vi "Initialize.vi"(8 "error in (no error)":errorcluster, 11 "State in":T1={"State"=enum."Idle", "Start Time"=timestamp(0 s since 1904-01-01), "Configuration"={"Cycle Period"=0.0, "PID 2 Parameters"={"Input Device"=enum."4-20mA", "Output Device"=enum."Default", "Setpoint"=0.0, "PID gains"={"proportional gain (Kc)"=0.0, "integral time (Ti, min)"=0.0, "derivative time (Td, min)"=100.0}, "output range"={"output low"=0.0, "output high"=1.0}}, "Manual Entry"=0.0, "Auto?"=TRUE, "4-20mA Input Settings"={"Input Channel "=0}, "4-20mA Out Settings"={"Output DAQ Task"=""}, "Input Channel Tag Name "=""}, "Current Time"=timestamp(0 s since 1904-01-01), "PID 1 Parameters"={"Setpoint"=0.0, "PID gains"={"proportional gain (Kc)"=1.0, "integral time (Ti, min)"=0.01, "derivative time (Td, min)"=0.0}}, "First Iteration"=FALSE, "Data"={"4-20mA Input"=0.0, "PID 2 Process Variable"=0.0, "PID 2 Output"=0.0, "4-20mA Output"=0.0}, "Process Name"="", "Pump On?"=enum."Off", "Input Error"=FALSE, "Output Error"=FALSE, "Log Started"=FALSE, "Current Setpoint"=0.0} {"Configuration"."PID 2 Parameters"."output range"."output low" format="%.2f"; "Configuration"."PID 2 Parameters"."output range"."output high" min=0.0 max=100.0 format="%.2f"; "Configuration"."PID 2 Parameters"."PID gains"."derivative time (Td, min)" format="%.3f"; "Configuration"."PID 2 Parameters"."PID gains"."integral time (Ti, min)" format="%.3f"; "Configuration"."PID 2 Parameters"."PID gains"."proportional gain (Kc)" format="%.3f"; "PID 1 Parameters"."PID gains"."derivative time (Td, min)" format="%.3f"; "PID 1 Parameters"."PID gains"."integral time (Ti, min)" format="%.3f"; "PID 1 Parameters"."PID gains"."proportional gain (Kc)" format="%.3f"}) -> (0 "error out":errorcluster, 1 "Pump Initialized":bool, 3 "State out":T1={"State"=enum."Idle", "Start Time"=timestamp(0 s since 1904-01-01), "Configuration"={"Cycle Period"=0.0, "PID 2 Parameters"={"Input Device"=enum."4-20mA", "Output Device"=enum."Default", "Setpoint"=0.0, "PID gains"={"proportional gain (Kc)"=0.0, "integral time (Ti, min)"=0.0, "derivative time (Td, min)"=100.0}, "output range"={"output low"=0.0, "output high"=1.0}}, "Manual Entry"=0.0, "Auto?"=TRUE, "4-20mA Input Settings"={"Input Channel "=0}, "4-20mA Out Settings"={"Output DAQ Task"=""}, "Input Channel Tag Name "=""}, "Current Time"=timestamp(0 s since 1904-01-01), "PID 1 Parameters"={"Setpoint"=0.0, "PID gains"={"proportional gain (Kc)"=1.0, "integral time (Ti, min)"=0.01, "derivative time (Td, min)"=0.0}}, "First Iteration"=FALSE, "Data"={"4-20mA Input"=0.0, "PID 2 Process Variable"=0.0, "PID 2 Output"=0.0, "4-20mA Output"=0.0}, "Process Name"="", "Pump On?"=enum."Off", "Input Error"=FALSE, "Output Error"=FALSE, "Log Started"=FALSE, "Current Setpoint"=0.0} {"Configuration"."PID 2 Parameters"."output range"."output low" format="%.2f"; "Configuration"."PID 2 Parameters"."output range"."output high" min=0.0 max=100.0 format="%.2f"; "Configuration"."PID 2 Parameters"."PID gains"."derivative time (Td, min)" format="%.3f"; "Configuration"."PID 2 Parameters"."PID gains"."integral time (Ti, min)" format="%.3f"; "Configuration"."PID 2 Parameters"."PID gains"."proportional gain (Kc)" format="%.3f"; "PID 1 Parameters"."PID gains"."derivative time (Td, min)" format="%.3f"; "PID 1 Parameters"."PID gains"."integral time (Ti, min)" format="%.3f"; "PID 1 Parameters"."PID gains"."proportional gain (Kc)" format="%.3f"})   [LabVIEW 2018, in "4-20mA Module.lvlib" / "4-20mA Module Engine.lvlib"]
uses:
  4-20mA Module Engine.lvlib
  State Cluster.ctl
  State Enum.ctl
  Pressure Transmitter/Pressure Transmitter Device Settings.ctl
  Pressure Reg Module/Pressure Regulator Device Settings.ctl
  Measure Instrument/PID 1 Parameters Cluster.ctl
  Tag VIs/Tag FGV Operation Enum.ctl
  Shared Variables/Dynamic Shared Variables.lvlib
  Pressure Transmitter/Pressure Transmitter Library.lvlib
  Pressure Reg Module/Pressure Regulator Library.lvlib
panel:
  # "Instrument Settings"
  # "Instrument Settings"
  # "Instrument Settings"
  # "Instrument Settings"
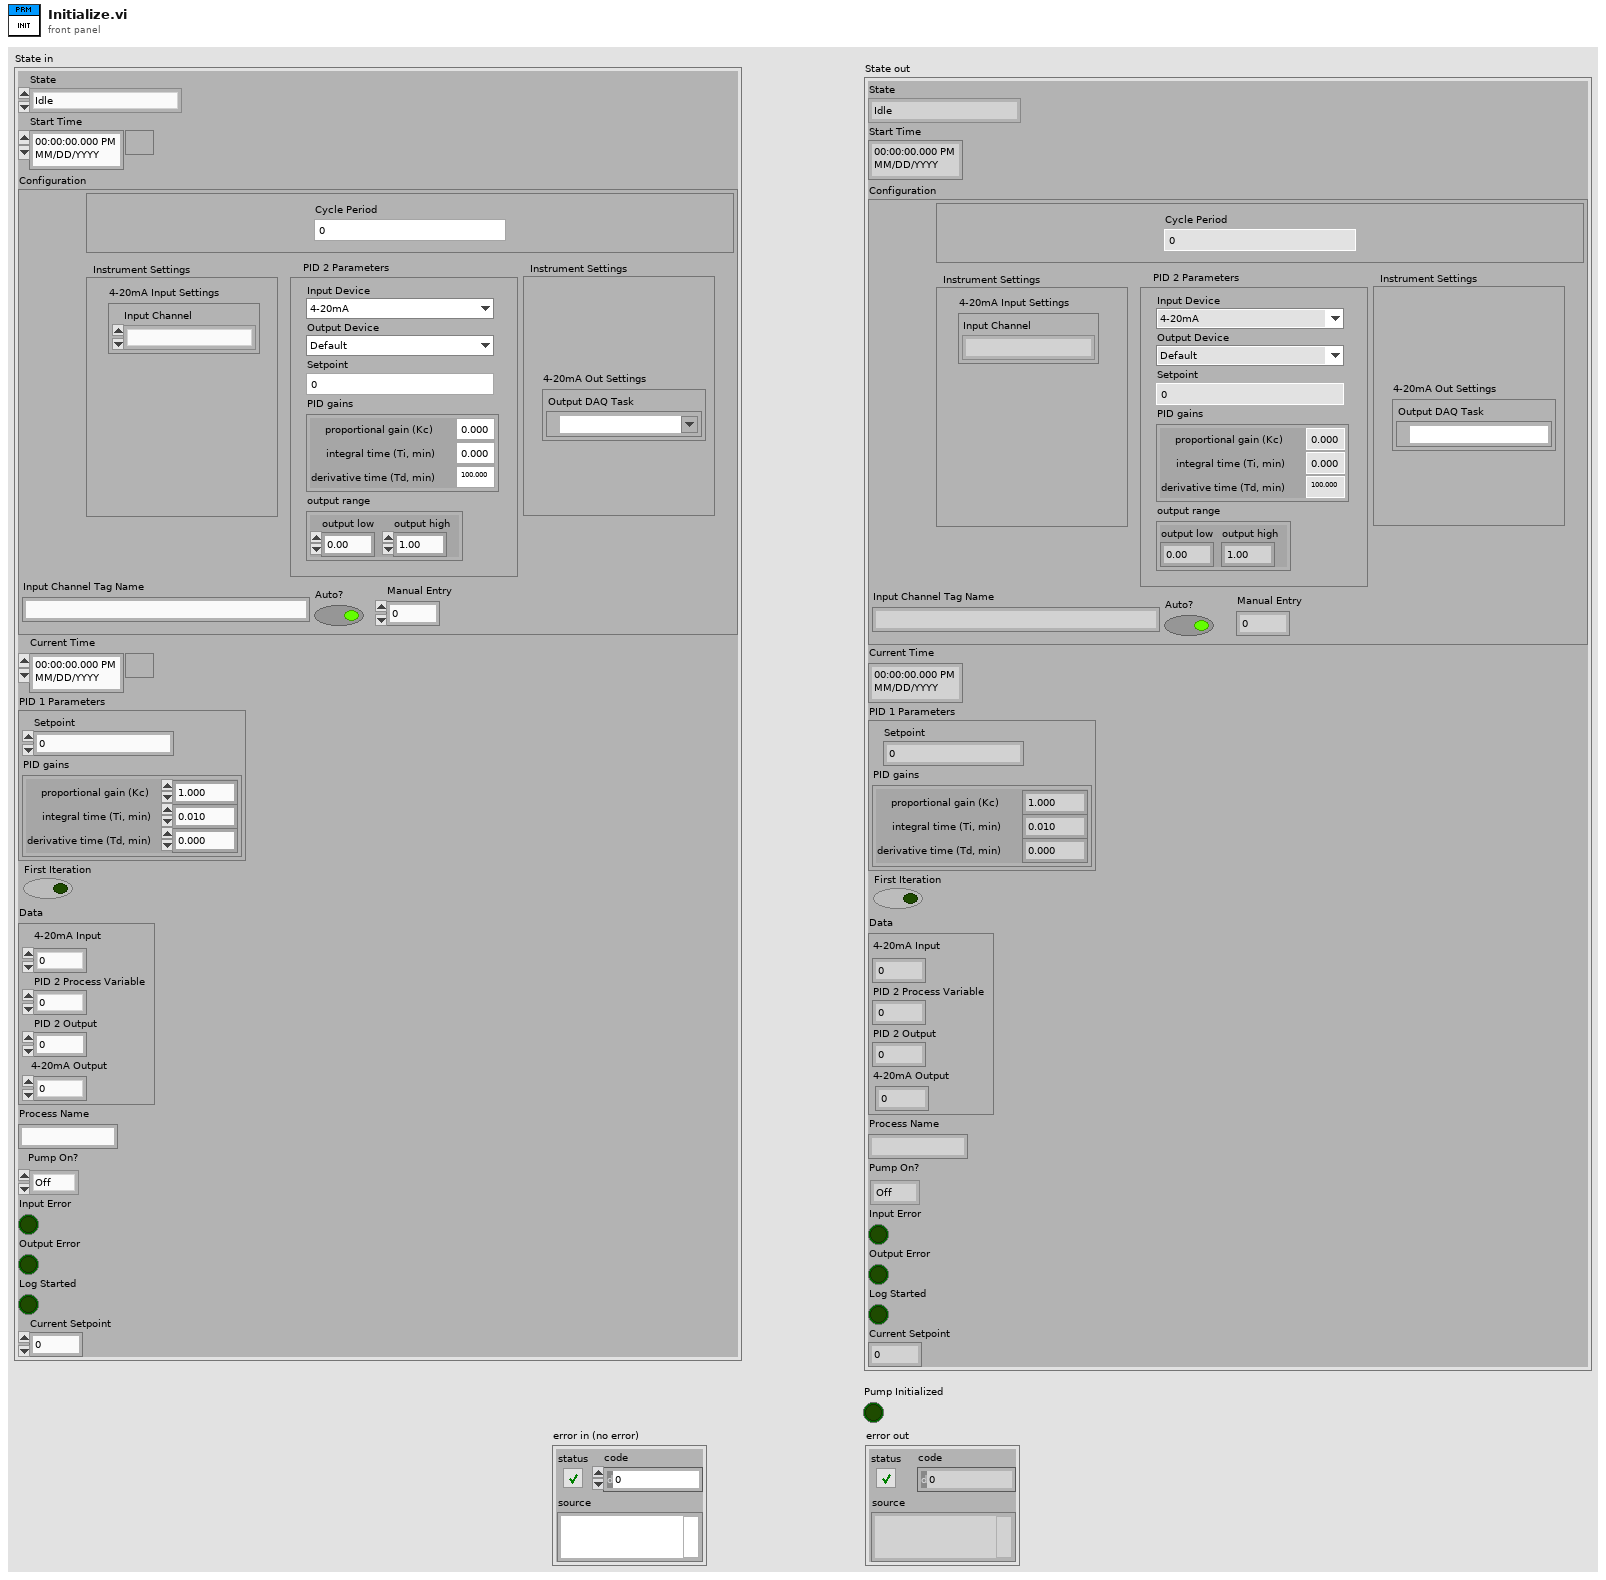
[diagram p1: front panel]
types:
  T1 = typedef "4-20mA Module.lvlib/4-20mA Module Engine.lvlib/State Cluster.ctl" = cluster{"State":T2, "Start Time":timestamp, "Configuration":cluster{"Cycle Period":dbl, "PID 2 Parameters":cluster{"Input Device":enum16{"Default", "4-20mA"}, "Output Device":enum16{"Default", "Equilibar Pressure Reg", "Flow Regulator"}, "Setpoint":dbl, "PID gains":cluster{"proportional gain (Kc)":dbl, "integral time (Ti, min)":dbl, "derivative time (Td, min)":dbl}, "output range":cluster{"output low":dbl, "output high":dbl}}, "Manual Entry":dbl, "Auto?":bool, "4-20mA Input Settings":T3, "4-20mA Out Settings":T4, "Input Channel Tag Name ":string}, "Current Time":timestamp, "PID 1 Parameters":T5, "First Iteration":bool, "Data":cluster{"4-20mA Input":dbl, "PID 2 Process Variable":dbl, "PID 2 Output":dbl, "4-20mA Output":dbl}, "Process Name":string, "Pump On?":enum16{"Off", "On", "Not Initialized"}, "Input Error":bool, "Output Error":bool, "Log Started":bool, "Current Setpoint":dbl}
  T2 = typedef "4-20mA Module.lvlib/4-20mA Module Engine.lvlib/State Enum.ctl" = enum16{"Measuring", "Idle", "Paused"}
  T3 = typedef "Pressure Transmitter Library.lvlib/Pressure Transmitter Device Settings.ctl" = cluster{"Input Channel ":u16}
  T4 = typedef "Pressure Regulator Library.lvlib/Pressure Regulator Device Settings.ctl" = cluster{"Output DAQ Task":refnum<k21>}
  T5 = typedef "PID 1 Parameters Cluster.ctl" = cluster{"Setpoint":dbl, "PID gains":cluster{"proportional gain (Kc)":dbl, "integral time (Ti, min)":dbl, "derivative time (Td, min)":dbl}}
  T6 = typedef "Tag FGV Operation Enum.ctl" = enum16{"Init", "Set Notification Queue", "Create Tag", "Commit", "Write Tag (Numeric)", "Write Tag (Boolean)", "Read All Tags", "Read One Tag", "Delete Tag Category", "Set Alarm Parameters (Numeric)", "Set Alarm Parameters (Boolean)", "Enable All Alarms", "Disable All Alarms", "Delete All Tags", "Read Alarms", "Ack Alarm", "Read Alarm Parameters (Numeric)", "Read Alarm Parameters (Boolean)"}
  T7 = typedef "4-20mA Module.lvlib/4-20mA Module Tag Names Cluster.ctl" = cluster{"4-20mA Input":string, "PID 2 Out Tag":string, "4-20mA Output":string, "Input Device Tag":string, "Output Device Tag":string}
  T8 = enum16{"Default", "Equilibar Pressure Reg", "Flow Regulator"}
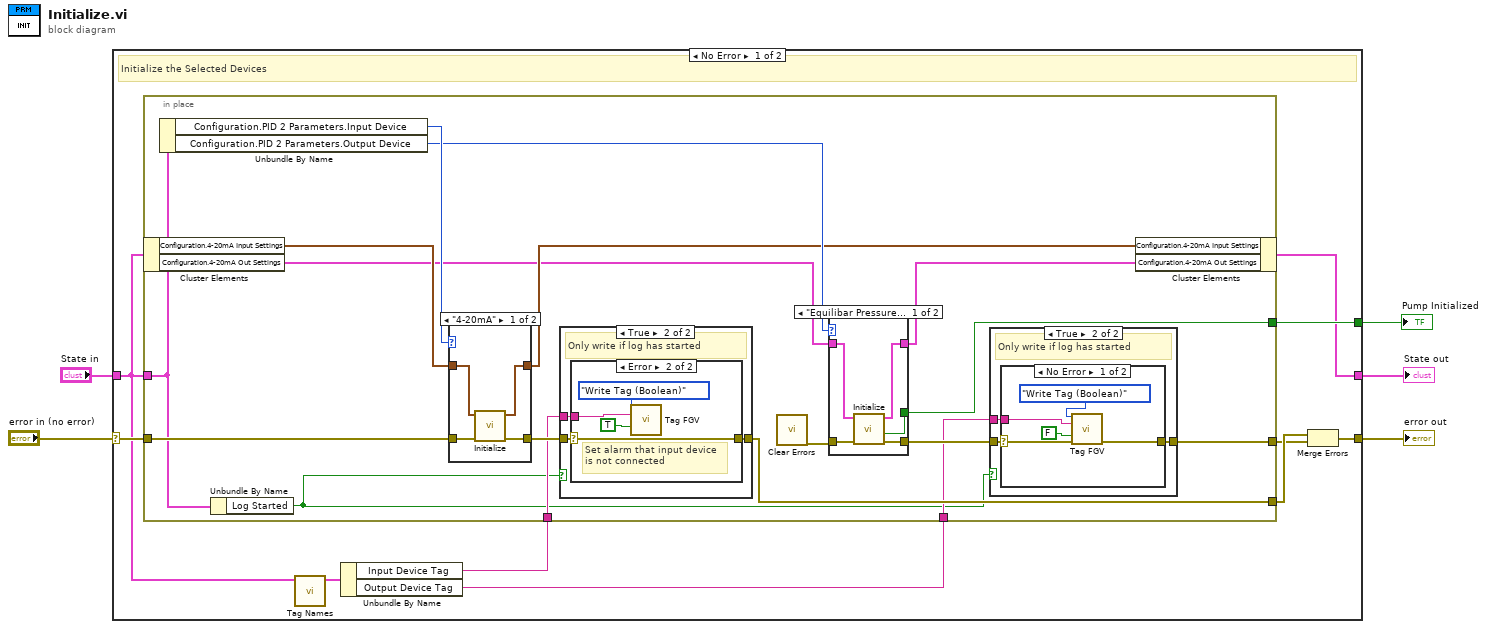
[diagram p0: block diagram]
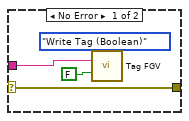
[diagram p3: hidden frame]
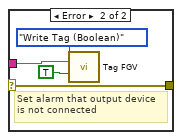
[diagram p5: hidden frame]
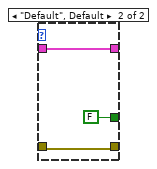
[diagram p6: hidden frame]
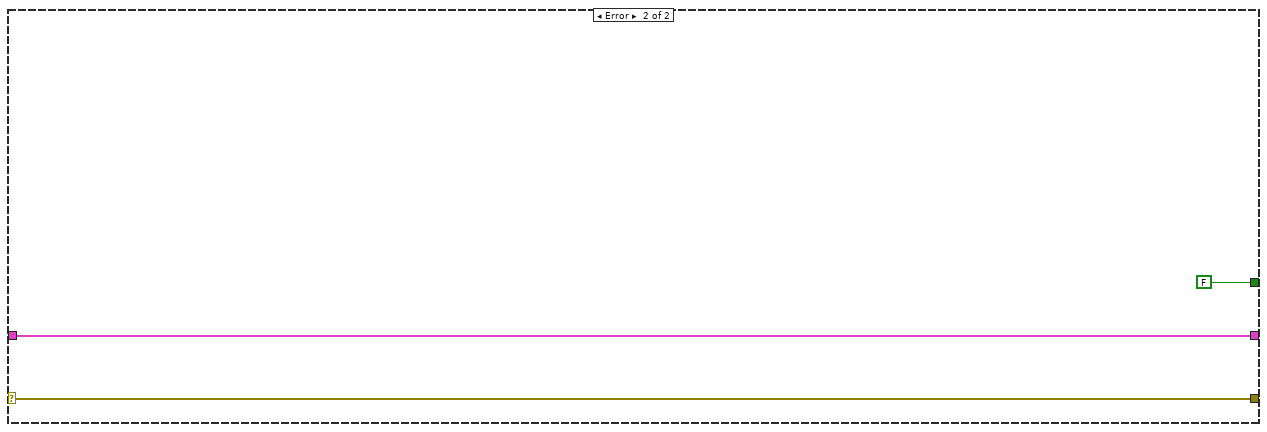
[diagram p8: hidden frame]
diagram:
  n1 = case shown="No Error" "error in (no error)" {
    selector: "error in (no error)" -> [w15 w74]
    tunnel: [w11 w74] -> w4
    tunnel: "State in" -> [w7 w73]
    tunnel: [w6 w73] -> w2
    tunnel: [w8 FALSE ("Initialized")] -> w1
    frame No Error {
      # "Initialize the Selected Devices"
      n2 = call "Tag Names.vi"("State in"=w7) -> ("4-20mA Module Tag Names"=w14:T7)  [unwired: 8 in, 2 out]
      n3 = Unbundle By Name(w14) -> ("Input Device Tag"=w13:string, "Output Device Tag"=w9:string)
      n4 = in-place {
        in-place-border: w15 -> [w31]
        in-place-border: w13 -> [w29]
        in-place-border: [w28] -> w12
        in-place-border: [w25] -> w10
        in-place-border: w9 -> [w24]
        in-place-border: [w22] -> w8
        in-place-border: w7 -> [w20]
        n5 = in-place-cluster #1(w7) -> ("Configuration.4-20mA Input Settings"=w17:T3, "Configuration.4-20mA Out Settings"=w16:T4)
        n6 = Unbundle By Name(w20) -> ("Configuration.PID 2 Parameters.Input Device"=w32:enum16{"Default", "4-20mA"}, "Configuration.PID 2 Parameters.Output Device"=w23:T8)
        n7 = Unbundle By Name(w20) -> ("Log Started"=w21:bool)
        n8 = case shown="\"4-20mA\"" w32 {
          tunnel: w17 -> [w67 w71]
          tunnel: w31 -> [w69 w70]
          tunnel: [w68 w70] -> w30
          tunnel: [w66 w71] -> w19
          frame "4-20mA" {
            n9 = call "Initialize.vi"("error in"=w69, "4-20mA Settings In"=w67) -> ("error out"=w68:errorcluster, "4-20mA Settings Out"=w66:T3)  [unwired: 7 in, 1 out]
          }
          frame "Default", Default {
          }
        }
        n10 = case shown="True" w21 {
          tunnel: w30 -> [w33 w36]
          tunnel: w29 -> [_ w35]
          tunnel: [w33 w34] -> w28
          frame False {
          }
          frame True {
            # "Only write if log has started"
            n11 = case shown="Error" w36 {
              selector: w36 -> [w37 w42]
              tunnel: [w37 w42] -> w34
              tunnel: w35 -> [w38 w41]
              frame No Error {
                n12 = call "Tag FGV.vi"("Operation"=Tag_FGV_Operation_Enum."Write Tag (Boolean)", "Tag Name"=w38, "Data"=FALSE) -> ()  [unwired: 5 in, 8 out]
              }
              frame Error {
                # "Set alarm that input device\nis not connected"
                n13 = call "Tag FGV.vi"("Operation"=Tag_FGV_Operation_Enum."Write Tag (Boolean)", "Tag Name"=w41, "Data"=TRUE) -> ()  [unwired: 5 in, 8 out]
              }
            }
          }
        }
        n14 = call <vilib>:"Clear Errors.vi"() -> ("error out"=w27:errorcluster)  [unwired: 6 in, 1 out]
        n15 = case shown="\"Equilibar Pressure Reg\"" w23 {
          tunnel: w16 -> [w59 w65]
          tunnel: [w58 w65] -> w18
          tunnel: w27 -> [w62 w64]
          tunnel: [w61 w64] -> w26
          tunnel: [w60 FALSE ("Initialized")] -> w22
          frame "Equilibar Pressure Reg" {
            n16 = call "Initialize.vi"("error in"=w62, "4-20mA Out Settings In"=w59) -> ("error out"=w61:errorcluster, "Initialized"=w60:bool, "4-20mA Out Settings Out"=w58:T4)  [unwired: 7 in]
          }
          frame "Default", Default {
          }
        }
        n17 = case shown="True" w21 {
          tunnel: w26 -> [w45 w48]
          tunnel: [w45 w47] -> w25
          tunnel: w24 -> [_ w46]
          frame False {
          }
          frame True {
            # "Only write if log has started"
            n18 = case shown="No Error" w48 {
              selector: w48 -> [w50 w55]
              tunnel: [w49 w55] -> w47
              tunnel: w46 -> [w51 w54]
              frame No Error {
                n19 = call "Tag FGV.vi"("Operation"=Tag_FGV_Operation_Enum."Write Tag (Boolean)", "Tag Name"=w51, "Data"=FALSE, "error in (no error)"=w50) -> ("error out"=w49:errorcluster)  [unwired: 4 in, 7 out]
              }
              frame Error {
                # "Set alarm that output device\nis not connected"
                n20 = call "Tag FGV.vi"("Operation"=Tag_FGV_Operation_Enum."Write Tag (Boolean)", "Tag Name"=w54, "Data"=TRUE) -> ()  [unwired: 5 in, 8 out]
              }
            }
          }
        }
        n21 = in-place-cluster #1("Configuration.4-20mA Input Settings"=w19, "Configuration.4-20mA Out Settings"=w18) -> (w6:T1)
      }
      n22 = Merge Errors(w12, w10) -> (w11:errorcluster)
    }
    frame Error {
    }
  }
  "error out" <- w4
  "State out" <- w2
  "Pump Initialized" <- w1
